vi "Generate Data Tables.vi"(0 "LBCB Number":T1, 2 "Cartesian Type":bool) -> (5 "Actuator Table":dbl[][](array[numeric]), 6 "Cartesian Table":dbl[][](array[numeric]))   [LabVIEW 2009]
uses:
  Data Access Objects/Metadata/LBCB Number.ctl
  Global Data/Actuator Measurment Actions.ctl
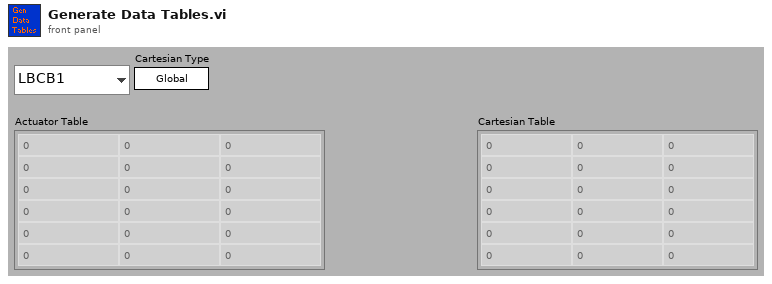
[diagram p1: front panel]
types:
  T1 = typedef "LBCB Number.ctl" = enum16{"LBCB1", "LBCB2"}
  T2 = typedef "Actuator Measurment Actions.ctl" = enum16{"Set  Data", "Get", "Init"}
  T3 = typedef "Cartesian Data Type.ctl" = cluster{"Displacements":dbl[], "Forces":dbl[], "Displacement Commands":dbl[]}
  T4 = typedef "Actuator DataType.ctl" = cluster{"LVDTs":dbl[], " Commands":dbl[], "Load Cells":dbl[], "Servo":dbl[]}
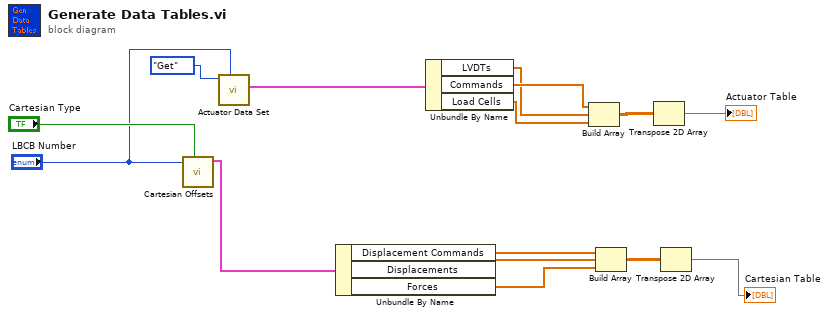
[diagram p0: block diagram]
diagram:
  n1 = call "Cartesian Offsets.vi"("Use Offsets"="Cartesian Type", "LBCB Number"="LBCB Number") -> ("Cartesian Data Out"=w3:T3)  [unwired: 7 out]
  n2 = call "Actuator Data Set.vi"("Selected LBCB"="LBCB Number", "Measurement Actions"=Actuator_Measurment_Actions."Get") -> ("Actuator Data Out"=w1:T4)  [unwired: 3 in, 6 out]
  n3 = Unbundle By Name(w3) -> ("Displacement Commands"=w9:dbl[], "Displacements"=w8:dbl[], "Forces"=w7:dbl[])
  n4 = Unbundle By Name(w1) -> ("LVDTs"=w11:dbl[], "Commands"=w12:dbl[], "Load Cells"=w13:dbl[])
  n5 = Build Array(w12, w11, w13) -> (w10:dbl[][])
  n6 = Build Array(w9, w8, w7) -> (w6:dbl[][])
  n7 = Transpose 2D Array(2D array=w10) -> (transposed array=→"Actuator Table":dbl[][])
  n8 = Transpose 2D Array(2D array=w6) -> (transposed array=→"Cartesian Table":dbl[][])
